vi "Set Absolute Time.vi"(8 "error in (no error)":errorcluster, 10 "System Time":T1={"Year"=1970, "Month"=1, "Day"=1, "Hours"=0, "Minutes"=0, "Seconds"=0} {"Seconds" min=0 max=60 step=1; "Minutes" min=0 max=60 step=1; "Hours" min=0 max=23 step=1; "Day" min=1 max=31 step=1; "Month" min=1 max=12 step=1; "Year" min=1970 step=1}, 11 "VISA resource name":refnum<visa-resource-name>) -> (0 "error out":errorcluster, 3 "VISA resource name out":refnum<visa-resource-name>)   [LabVIEW 2021, in "Keithley 2450.lvlib"]
doc: "This sets the absolute time of the instrument."
uses:
  Keithley 2450.lvlib
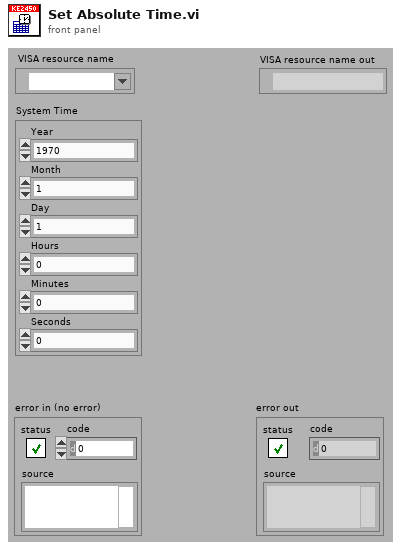
[diagram p1: front panel]
types:
  T1 = cluster{"Year":i32, "Month":i32, "Day":i32, "Hours":i32, "Minutes":i32, "Seconds":i32}
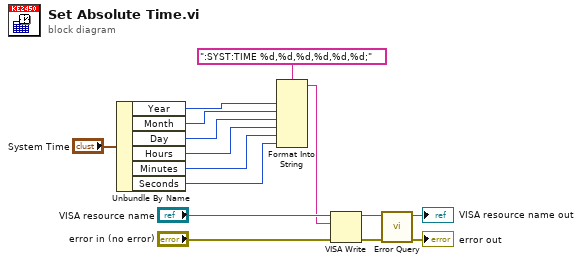
[diagram p0: block diagram]
diagram:
  n1 = Unbundle By Name("System Time") -> ("Year"=w6:i32, "Month"=w5:i32, "Day"=w4:i32, "Hours"=w3:i32, "Minutes"=w2:i32, "Seconds"=w1:i32)
  n2 = Format Into String(format string=":SYST:TIME %d,%d,%d,%d,%d,%d;", w6, w5, w4, w3, w2, w1) -> (resulting string=w9:string)  [unwired: 2 in, 1 out]
  n3 = VISA Write(VISA resource name="VISA resource name", write buffer=w9, error in (no error)="error in (no error)") -> (VISA resource name out=w11:refnum<visa-resource-name>, error out=w10:errorcluster)  [unwired: 1 out]
  n4 = call "Error Query.vi"("error in (no error)"=w10, "VISA resource name"=w11) -> ("error out"=→"error out":errorcluster, "VISA resource name out"=→"VISA resource name out":refnum<visa-resource-name>)  [unwired: 8 out]
